vi "Exercise 2.4 - Write to Spreadsheet File.vi"() -> ()   [LabVIEW 2024]
panel:
  in  "stop":bool
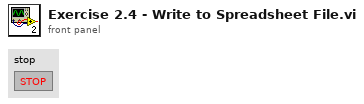
[diagram p1: front panel]
types:
  T1 = enum16{"open", "replace", "create", "open or create", "replace or create", "replace or create with confirmation"}
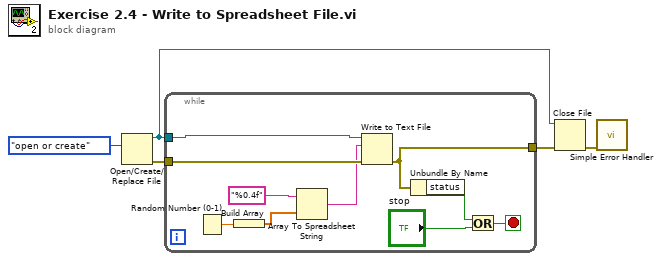
[diagram p0: block diagram]
diagram:
  n1 = Open/Create/Replace File(operation (0:open)=T1."open or create") -> (refnum out=w2:refnum<file>, error out=w4:errorcluster)  [unwired: 5 in, 1 out]
  n2 = while {
    tunnel: w2 -> [w15]
    tunnel: w4 -> [w14]
    tunnel: [w10] -> w3
    stop <- w9 stop-if-true
    n3 = Random Number (0-1)() -> (number: 0 to 1=w8:dbl)
    n4 = Build Array(w8) -> (w7:dbl[])
    n5 = Array To Spreadsheet String(array=w7, 3:"%0.4f" ("format string")) -> (spreadsheet string=w6:string)  [unwired: 1 in]
    n6 = Write to Text File(file (use dialog)=w15, text=w6, error in=w14) -> (error out=w10:errorcluster)  [unwired: 1 in, 2 out]
    n7 = Unbundle By Name(w10) -> ("status"=w12:bool)
    n8 = Or(x=w12, y="stop") -> (x .or. y?=w9:bool)
  }
  n9 = Close File(refnum=w2, error in=w3) -> (error out=w1:errorcluster)  [unwired: 1 out]
  n10 = call <vilib>:"Simple Error Handler.vi"("error in (no error)"=w1) -> ()  [unwired: 4 in, 5 out]
